vi "Write Polling Iterations.vi"(8 "error in (no error)":errorcluster, 10 "Polling Iterations":u32, 11 "Write Polling Iterations Msg in":refnum<class "Polling Iterations Msg.lvclass">) -> (0 "error out":errorcluster, 3 "Write Polling Iterations Msg out":refnum<class "Polling Iterations Msg.lvclass">)   [LabVIEW 2016, in "CS++BaseActor.lvlib" / "Polling Iterations Msg.lvclass"]
uses:
  Polling Iterations Msg.lvclass
  Polling Iterations Msg.lvclass/Polling Iterations Msg.ctl
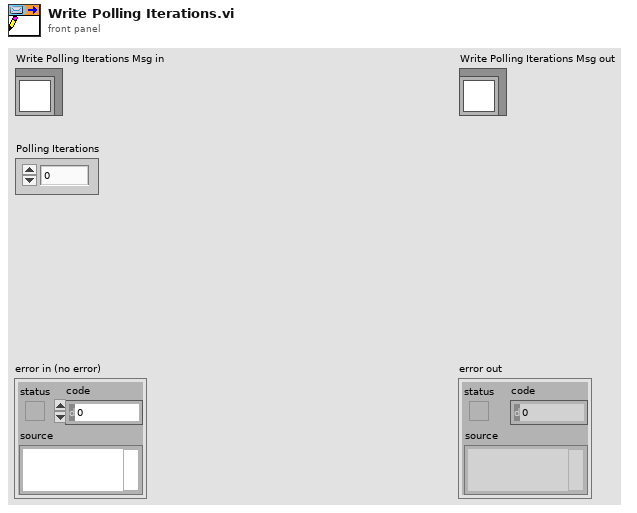
[diagram p1: front panel]
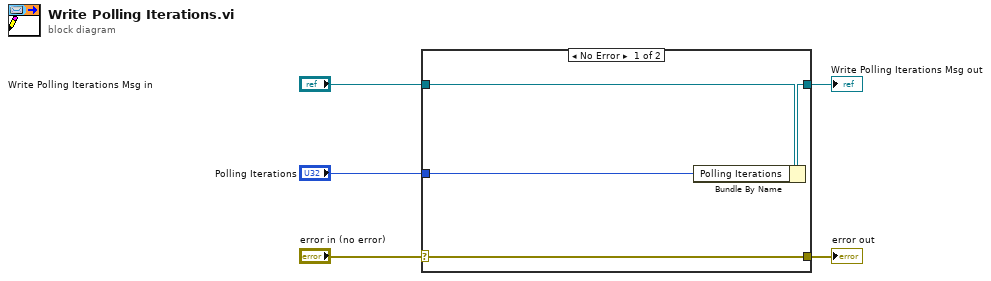
[diagram p0: block diagram]
diagram:
  n1 = case shown="No Error" "error in (no error)" {
    selector: "error in (no error)" -> [w9 w10]
    tunnel: [w9 w10] -> w4
    tunnel: [w7 w11] -> w2
    tunnel: "Write Polling Iterations Msg in" -> [w8 w11]
    tunnel: "Polling Iterations" -> [w6 _]
    frame No Error {
      n2 = Bundle By Name(cluster=w8, "Polling Iterations"=w6) -> (w7:refnum<class "Polling Iterations Msg.lvclass">)
    }
    frame Error {
    }
  }
  "error out" <- w4
  "Write Polling Iterations Msg out" <- w2
